vi "Encode_Data.vi"(0 "error in (no error)":errorcluster, 1 "Data In":string) -> (2 "error out":errorcluster, 3 "Data IN Device 1":string, 4 "Data IN Device 0":string)   [LabVIEW 2010]
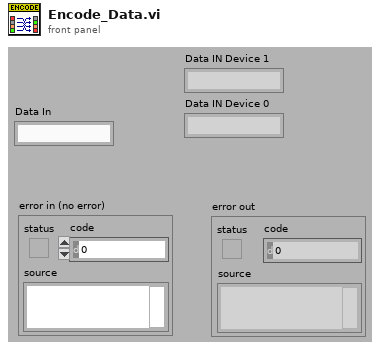
[diagram p1: front panel]
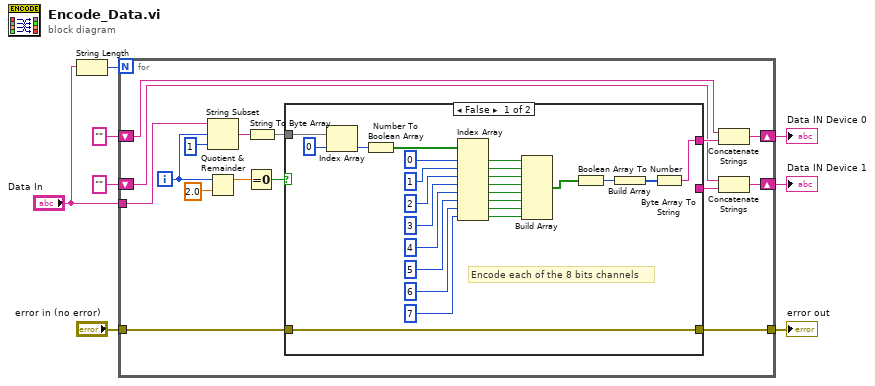
[diagram p0: block diagram]
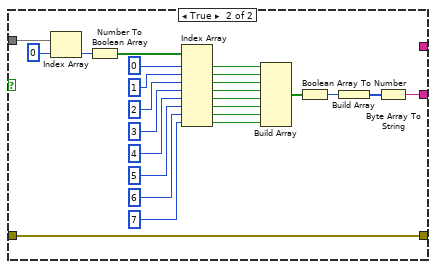
[diagram p2: hidden frame]
diagram:
  n1 = String Length(string="Data In") -> (length=w8:i32)
  n2 = for {
    N: w8 -> [_]
    tunnel: "Data In" -> [w24]
    shift-right: [w16] -> w6
    shift-left: "" -> [w12]
    shift-right: [w14] -> w5
    shift-left: "" -> [w11]
    tunnel: [w10] -> w2
    tunnel: "error in (no error)" -> [w9]
    i -> [w21]
    n3 = String Subset(string=w24, offset (0)=w21, length (rest)=1 ("length (rest)")) -> (substring=w17:string)
    n4 = Quotient & Remainder(x=w21, y=2.0) -> (x-y*floor(x/y)=w20:dbl)  [unwired: 1 out]
    n5 = Equal To 0?(x=w20) -> (x = 0?=w19:bool)
    n6 = String To Byte Array(string=w17) -> (unsigned byte array=w18:u8[])
    n7 = case shown="False" w19 {
      tunnel: w18 -> [w36 w56]
      tunnel: [_ w50] -> w15
      tunnel: [w25 _] -> w13
      tunnel: [w35 w55] -> w10
      tunnel: w9 -> [w35 w55]
      frame False {
        # "Encode each of the 8 bits channels"
        n8 = Index Array(array=w36, index=0) -> (element=w48:u8)
        n9 = Number To Boolean Array(number=w48) -> (Boolean array=w47:bool[])
        n10 = Index Array(array=w47, index #1=0 ("index"), index #2=1 ("index"), index #3=2 ("index"), index #4=3 ("index"), index #5=4 ("index"), index #6=5 ("index"), index #7=6 ("index"), index #8=7 ("index")) -> (element #1=w33:bool, element #2=w32:bool, element #3=w31:bool, element #4=w30:bool, element #5=w29:bool, element #6=w28:bool, element #7=w27:bool, element #8=w26:bool)
        n11 = Build Array(w33, w32, w31, w30, w29, w28, w27, w26) -> (w34:bool[])
        n12 = Boolean Array To Number(Boolean array=w34) -> (number=w38:u32)
        n13 = Build Array(w38) -> (w37:u32[])
        n14 = Byte Array To String(unsigned byte array=w37) -> (string=w25:string)
      }
      frame True {
        n15 = Index Array(array=w56, index=0) -> (element=w73:u8)
        n16 = Number To Boolean Array(number=w73) -> (Boolean array=w72:bool[])
        n17 = Index Array(array=w72, index #1=0 ("index"), index #2=1 ("index"), index #3=2 ("index"), index #4=3 ("index"), index #5=4 ("index"), index #6=5 ("index"), index #7=6 ("index"), index #8=7 ("index")) -> (element #1=w61:bool, element #2=w60:bool, element #3=w59:bool, element #4=w58:bool, element #5=w54:bool, element #6=w53:bool, element #7=w52:bool, element #8=w51:bool)
        n18 = Build Array(w61, w60, w59, w58, w54, w53, w52, w51) -> (w57:bool[])
        n19 = Boolean Array To Number(Boolean array=w57) -> (number=w63:u32)
        n20 = Build Array(w63) -> (w62:u32[])
        n21 = Byte Array To String(unsigned byte array=w62) -> (string=w50:string)
      }
    }
    n22 = Concatenate Strings(w11, w13) -> (w14:string)
    n23 = Concatenate Strings(w12, w15) -> (w16:string)
  }
  "Data IN Device 1" <- w6
  "Data IN Device 0" <- w5
  "error out" <- w2
